vi "main.vi"() -> ()   [LabVIEW 2019]
uses:
  <vilib>/Utility/sysdir.llb/System Directory Type.ctl
  <vilib>/Platform/browser.llb/Open URL in Default Browser (string).vi
  <vilib>/Utility/cursorutil.llb/Set Cursor (Icon Pict).vi
  <vilib>/regexp/Match Regular Expression.xnode
  lib/libSimulationControl/libSimulationControl.lvlib
panel:
  out "Impressum":string
  out "Running?":bool
  in  "Help Button":bool
  in  "Break":bool
  in  "Plot":bool
  in  "Stop Button":bool
  in  "Pause Button":bool
  in  "Run":bool
  in  "Tab Control":T1(tab)
  out "Active element":string
  out "Iteration":i32
  out "Plant structure":string
  out "Simulation log":string
  in  "Auto Scroll":bool
  in  "Reset":bool
  in  "Uncouple":bool
  out "Working directory":path
  out "Runtime":dbl
  in  "Console":bool
  out "Runtime":string
  in  "Env. Clear":bool
  out "Env. Structure":string
  in  "Load Env":bool
  out "Environtment ready?":bool
  in  "Create Env":bool
  in  "Environtment Dir":path
  in  "Environment Tree":string(tree)
  out "Reactor Legend":picture
  in  "Show legend":bool
  out "Feedback?":bool
  out "Methane?":bool
  out "Storage?":bool
  out "#Hydrolysis":dbl
  out "Plant":picture
  in  "Reactor State":string(combo)="STRUCT_1_STAGE.vi"
  in  "Hydrolysis specification":path
  in  "Methane specification":path
  in  "Auto cleanup?":bool
  in  "Endtime":dbl
  in  "Starttime":dbl
  in  "Edit Methane":bool
  in  "Edit Hydro":bool
  in  "Simulation file":path
  out "#Reactors":i32
  in  "Inflow fractions":T2(array[cluster]) {"Vertical Pointer Slide" scale=0.0..100.0 scale format="%.0f%"}
  in  "Hydrolysis PH":cluster{"Meter":dbl, "String":string}[][](array[cluster]) {"Meter" scale=0.0..14.0}
  in  "Load Feeding":bool
  in  "Save Feeding":bool
  out "Valid stamp?":bool
  out "Next timestep":dbl
  in  "Reactor":string(combo)
  in  "Delete":bool
  in  "Add timestamp":string[](array[string])
  in  "Add":bool
  in  "Feeding table":i32(listbox)
  out "timetable":string
  # "Biogas simulation Control"
  # "Before you start the simulation you need to set up a working environment.\nThe environment will be for the chosen reactor structure only."
  # "If you want the hydrolysis reactors to start with different initial values, you need to set up a working environtment first."
  # "Change the proportions at which the methane outflow will \nbe fed back into the hydrolysis reactors:"
  # "Add feeding hours and amount for a hydrolysis reactor."
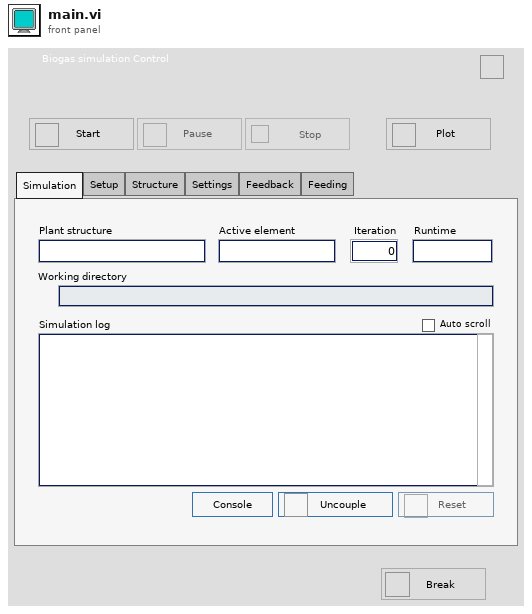
[diagram p1: front panel]
types:
  T1 = enum32{"Simulation", "Setup", "Structure", "Settings", "Feedback", "Feeding"}
  T2 = cluster{"Vertical Pointer Slide":i32, "String":string}[]
  T3 = typedef "System Directory Type.ctl" = i32
  T4 = enum8{"Enabled", "Disabled", "Disabled and Grayed Out"}
  T5 = typedef "LVPoint32TypeDef.ctl" = cluster{"Horizontal":i32, "Vertical":i32}
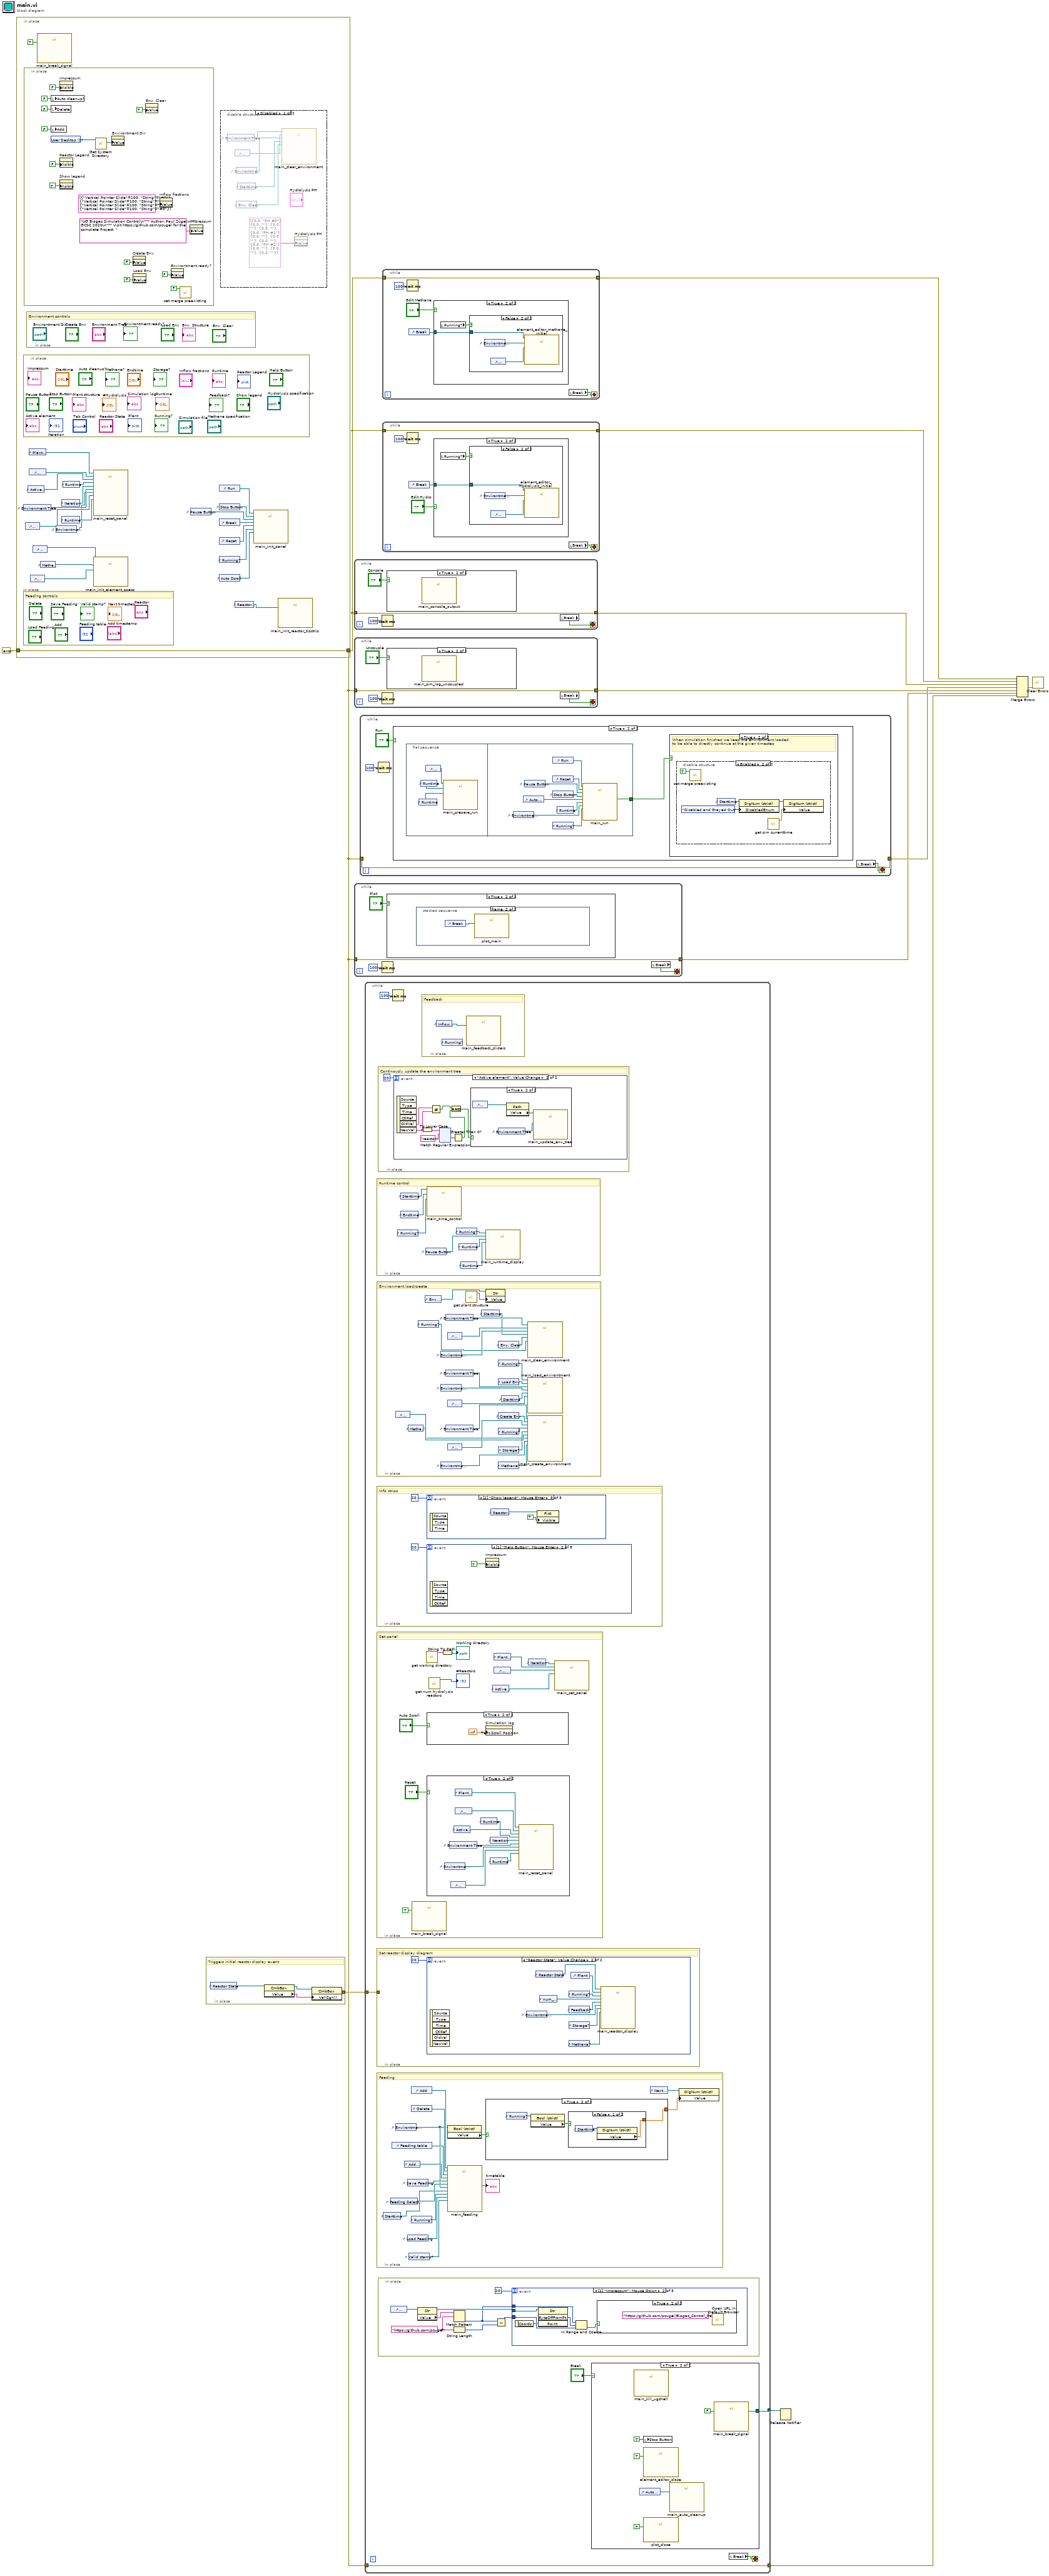
[diagram p0: block diagram]
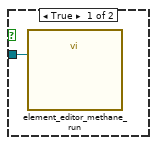
[diagram p3: hidden frame]
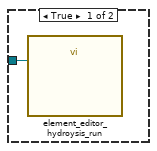
[diagram p5: hidden frame]
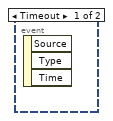
[diagram p8: hidden frame]
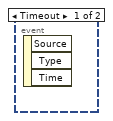
[diagram p10: hidden frame]
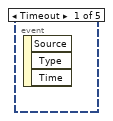
[diagram p11: hidden frame]
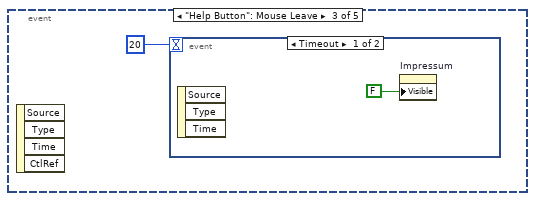
[diagram p12: hidden frame]
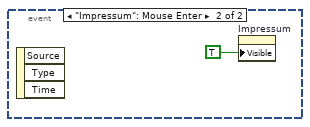
[diagram p13: hidden frame]
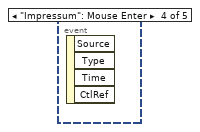
[diagram p14: hidden frame]
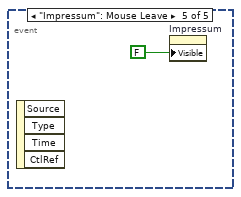
[diagram p15: hidden frame]
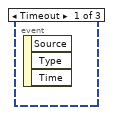
[diagram p16: hidden frame]
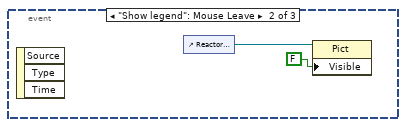
[diagram p17: hidden frame]
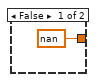
[diagram p20: hidden frame]
diagram:
  n1 = in-place {
    in-place-border: [w34] -> w5
    in-place-border: errorcluster {"status"=FALSE, "code"=0, "source"=""} ("error constant") -> [w34]
    n2 = in-place {
    }
    n3 = control-ref of="Environment Tree"() -> (w17:refnum<vi>)
    n4 = in-place {
      # "Feeding controls"
    }
    n5 = in-place {
      w46 = T3 1 items=["User Home"=0, "User Desktop"=1, "User Documents"=2, "User Application Data"=3, "User Preferences"=4, "User Temporary"=5, "Public Documents"=6, "Public Application Data"=7, "Public Preferences"=8, "Public Cache"=13, "System Core Libraries"=9, "System Installed Libraries"=10, "Application Files"=11, "Boot Volume Root"=12] ("system directory type")
      n6 = local write "Auto cleanup?"(FALSE ("Auto Cleanup?")) -> ()
      n7 = local write "Delete"(FALSE ("Delete")) -> ()
      n8 = local write "Add"(FALSE ("Add")) -> ()
      n9 = property on="Impressum" class="Str"("Visible"=FALSE) -> ()  [unwired: 2 in, 2 out]
      n10 = property on="Reactor Legend" class="Pict"("Visible"=FALSE) -> ()  [unwired: 2 in, 2 out]
      n11 = property on="Show legend" class="Bool"("Visible"=TRUE) -> ()  [unwired: 2 in, 2 out]
      n12 = call <vilib>:"Get System Directory.vi"("system directory type"=w46) -> ("system directory"=w47:path)  [unwired: 10 in]
      n13 = property on="Environtment Dir" class="Path"("Value"=w47) -> ()  [unwired: 2 in, 2 out]
      n14 = property on="Create Env" class="Bool (strict)"("Value"=FALSE ("Create Env")) -> ()  [unwired: 2 in, 2 out]
      n15 = property on="Load Env" class="Bool (strict)"("Value"=FALSE ("Load Env")) -> ()  [unwired: 2 in, 2 out]
      n16 = property on="Env. Clear" class="Bool (strict)"("Value"=TRUE ("Env. Clear")) -> ()  [unwired: 2 in, 2 out]
      n17 = property on="Inflow fractions" class="Arr (strict)"("Value"=T2 [{"Vertical Pointer Slide"=100, "String"="#0"}, {"Vertical Pointer Slide"=100, "String"="#1"}, {"Vertical Pointer Slide"=100, "String"="#2"}, {"Vertical Pointer Slide"=100, "String"="#3"}] ("Inflow fractions")) -> ()  [unwired: 2 in, 2 out]
      n18 = property on="Environtment ready?" class="Bool (strict)"("Value"=FALSE ("Environtment ready?")) -> ()  [unwired: 2 in, 2 out]
      n19 = call "set merge preexisting.vi"("merge"=FALSE) -> ()  [unwired: 10 in, 1 out]
      n20 = property on="Impressum" class="Str"("Value"="UG Biogas Simulation Control\n*** Author: Paul Zügel\n*** GCSC 2020\n*** Visit https://github.com/pzugel for the complete Project  " ("String")) -> ()  [unwired: 2 in, 2 out]
    }
    n21 = control-ref of="Environtment Dir"() -> (w18:refnum<vi>)
    n22 = in-place {
      # "Environment controls"
    }
    n23 = control-ref of="Active element"() -> (w32:refnum<vi>)
    n24 = control-ref of="Plant structure"() -> (w30:refnum<vi>)
    n25 = control-ref of="Simulation log"() -> (w31:refnum<vi>)
    n26 = control-ref of="Simulation file"() -> (w20:refnum<vi>)
    n27 = control-ref of="Hydrolysis specification"() -> (w14:refnum<vi>)
    n28 = call "main_break_signal.vi"("Keep Running?"=TRUE ("Checkbox")) -> ()  [unwired: 10 in, 1 out]
    n29 = control-ref of="Methane specification"() -> (w13:refnum<vi>)
    n30 = control-ref of="Environtment ready?"() -> (w16:refnum<vi>)
    n31 = control-ref of="Iteration"() -> (w33:refnum<vi>)
    n32 = control-ref of="Runtime"() -> (w21:refnum<vi>)
    n33 = control-ref of="Runtime"() -> (w19:refnum<vi>)
    n34 = call "main_reset_panel.vi"("Env ready?"=w16, "Envi. Tree"=w17, "Env. Directory"=w18, "Iteration"=w33, "Runtime"=w21, "Runtime (string)"=w19, "Active Element"=w32, "Simulation Log"=w31, "Plant Structure"=w30) -> ()  [unwired: 3 in]
    n35 = call "main_init_element_specs.vi"("Simulation"=w20, "Methane"=w13, "Hydrolyse"=w14) -> ()  [unwired: 9 in]
    n36 = control-ref of="Pause Button"() -> (w23:refnum<vi>)
    n37 = control-ref of="Run"() -> (w29:refnum<vi>)
    n38 = control-ref of="Stop Button"() -> (w24:refnum<vi>)
    n39 = control-ref of="Break"() -> (w27:refnum<vi>)
    n40 = control-ref of="Reset"() -> (w28:refnum<vi>)
    n41 = control-ref of="Running?"() -> (w22:refnum<vi>)
    n42 = control-ref of="Auto Scroll"() -> (w26:refnum<vi>)
    n43 = disable-structure shown="Disabled" {
      frame Disabled {
        n44 = control-ref of="Environment Tree"() -> (w40:refnum<vi>)
        n45 = control-ref of="Environtment Dir"() -> (w39:refnum<vi>)
        n46 = control-ref of="Environtment ready?"() -> (w38:refnum<vi>)
        n47 = control-ref of="Env. Clear"() -> (w36:refnum<vi>)
        n48 = control-ref of="Starttime"() -> (w37:refnum<vi>)
        n49 = call "main_clear_environment.vi"("Env. Clear"=w36, "Starttime"=w37, "Env. ready?"=w38, "Env. Dir"=w39, "Env. Tree"=w40) -> ()  [unwired: 7 in]
        n50 = property on="Hydrolysis PH" class="Arr (strict)"("Value"=cluster{"Meter":dbl, "String":string}[][] [[{"Meter"=0.0, "String"="PH #0"}, {"Meter"=0.0, "String"=""}, {"Meter"=0.0, "String"=""}, {"Meter"=0.0, "String"=""}], [{"Meter"=0.0, "String"="PH #1"}, {"Meter"=0.0, "String"=""}, {"Meter"=0.0, "String"=""}, {"Meter"=0.0, "String"=""}], [{"Meter"=0.0, "String"="PH #2"}, {"Meter"=0.0, "String"=""}, {"Meter"=0.0, "String"=""}, {"Meter"=0.0, "String"=""}]] ("Hydrolysis PH")) -> ()  [unwired: 2 in, 2 out]
      }
      frame Enabled {
      }
    }
    n51 = control-ref of="Reactor Legend"() -> (w15:refnum<vi>)
    n52 = call "main_init_panel.vi"("Running?"=w22, "Reset"=w28, "Auto Scroll"=w26, "Break Button"=w27, "Pause Button"=w23, "Stop Button"=w24, "Run"=w29) -> ()  [unwired: 5 in]
    n53 = call "main_init_reactor_tipstrip.vi"("Reactor legend"=w15) -> ()  [unwired: 11 in]
  }
  n54 = in-place {
    in-place-border: [w56] -> w1
    # "Triggers initial reactor display event"
    n55 = control-ref of="Reactor State"() -> (w59:refnum<vi>)
    n56 = property class="CmbBox"(reference=w59) -> (reference out=w57:refnum<vi>, "Value"=w58:string)  [unwired: 1 in, 1 out]
    n57 = property class="CmbBox"(reference=w57, "Val(Sgnl)"=w58) -> (error out=w56:errorcluster)  [unwired: 1 in, 1 out]
  }
  n58 = while {
    tunnel: w5 -> [w62]
    tunnel: [w62] -> w6
    stop <- w60 stop-if-true
    n59 = Wait (ms)(milliseconds to wait=u32 100) -> ()  [unwired: 1 out]
    n60 = case shown="True" "Console" {
      frame False {
      }
      frame True {
        n61 = call "main_console_output.vi"() -> ()  [unwired: 12 in]
      }
    }
    n62 = local read "Break"() -> (w60:bool)
  }
  n63 = while {
    tunnel: w5 -> [w66]
    tunnel: [w66] -> w7
    stop <- w64 stop-if-true
    n64 = Wait (ms)(milliseconds to wait=u32 100) -> ()  [unwired: 1 out]
    n65 = case shown="True" "Uncouple" {
      frame False {
      }
      frame True {
        n66 = call "main_sim_log_uncoupled.vi"() -> ()  [unwired: 12 in]
      }
    }
    n67 = local read "Break"() -> (w64:bool)
  }
  n68 = while {
    tunnel: w5 -> [w70]
    tunnel: [w70] -> w10
    stop <- w68 stop-if-true
    n69 = Wait (ms)(milliseconds to wait=u32 100) -> ()  [unwired: 1 out]
    n70 = case shown="True" "Plot" {
      frame False {
      }
      frame True {
        n71 = stacked-sequence {
          frame #0 {
            n72 = call "plot_close.vi"("Close?"=TRUE) -> ()  [unwired: 11 in]
          }
          frame #1 {
            n73 = control-ref of="Break"() -> (w73:refnum<vi>)
            n74 = call "plot_main.vi"("Break"=w73) -> ()  [unwired: 11 in]
          }
        }
      }
    }
    n75 = local read "Break"() -> (w68:bool)
  }
  n76 = while {
    tunnel: w5 -> [w77]
    tunnel: [w77] -> w11
    stop <- w75 stop-if-true
    n77 = Wait (ms)(milliseconds to wait=u32 100) -> ()  [unwired: 1 out]
    n78 = case shown="True" "Run" {
      frame False {
        n79 = property on="Run" class="Bool"("DisabledEnum"=T4."Enabled" ("Disabled")) -> ()  [unwired: 2 in, 2 out]
        n80 = property on="Stop Button" class="Bool (strict)"("DisabledEnum"=T4."Disabled and Grayed Out" ("Disabled")) -> ()  [unwired: 2 in, 2 out]
        n81 = property on="Pause Button" class="Bool (strict)"("DisabledEnum"=T4."Disabled and Grayed Out" ("Disabled")) -> ()  [unwired: 2 in, 2 out]
      }
      frame True {
        n82 = flat-sequence {
          tunnel: [w96] -> w81
          frame #0 {
            n83 = control-ref of="Runtime"() -> (w95:refnum<vi>)
            n84 = control-ref of="Runtime"() -> (w94:refnum<vi>)
            n85 = control-ref of="Environtment Dir"() -> (w93:refnum<vi>)
            n86 = call "main_prepare_run.vi"("Runtime"=w95, "Runtime String"=w94, "Env. Dir"=w93) -> ()  [unwired: 9 in]
          }
          frame #1 {
            n87 = control-ref of="Environtment ready?"() -> (w104:refnum<vi>)
            n88 = control-ref of="Auto cleanup?"() -> (w103:refnum<vi>)
            n89 = control-ref of="Pause Button"() -> (w100:refnum<vi>)
            n90 = control-ref of="Run"() -> (w98:refnum<vi>)
            n91 = control-ref of="Reset"() -> (w102:refnum<vi>)
            n92 = control-ref of="Stop Button"() -> (w99:refnum<vi>)
            n93 = control-ref of="Running?"() -> (w101:refnum<vi>)
            n94 = control-ref of="Runtime"() -> (w97:refnum<vi>)
            n95 = call "main_run.vi"("Runtime String"=w97, "Env ready?"=w104, "Cleanup?"=w103, "Running?"=w101, "Stop Button"=w99, "Pause Button"=w100, "Reset"=w102, "Run"=w98) -> ("OK?"=w96:bool)  [unwired: 3 in]
          }
        }
        n96 = case shown="True" w81 {
          frame False {
          }
          frame True {
            # "When simulation finished we keep the environment loaded\nto be able to directly continue at the given timestep"
            n97 = disable-structure shown="Enabled" {
              frame Disabled {
                n98 = control-ref of="Env. Clear"() -> (w86:refnum<vi>)
                n99 = property class="Bool (strict)"(reference=w86, "Value"=TRUE) -> (reference out=w87:refnum<vi>)  [unwired: 1 in, 1 out]
                n100 = control-ref of="Environtment ready?"() -> (w85:refnum<vi>)
                n101 = control-ref of="Environment Tree"() -> (w83:refnum<vi>)
                n102 = control-ref of="Environtment Dir"() -> (w84:refnum<vi>)
                n103 = call "main_clear_environment.vi"("Env. Clear"=w87, "Env. ready?"=w85, "Env. Dir"=w84, "Env. Tree"=w83) -> ()  [unwired: 8 in]
              }
              frame Enabled {
                n104 = call "set merge preexisting.vi"("merge"=TRUE) -> ()  [unwired: 10 in, 1 out]
                n105 = control-ref of="Starttime"() -> (w91:refnum<vi>)
                n106 = property class="DigNum (strict)"(reference=w91, "DisabledEnum"=T4."Disabled and Grayed Out" ("Disabled")) -> (reference out=w88:refnum<vi>)  [unwired: 1 in, 1 out]
                n107 = call "get sim currenttime.vi"() -> ("current_time"=w89:dbl)  [unwired: 10 in, 1 out]
                n108 = property class="DigNum (strict)"(reference=w88, "Value"=w89) -> ()  [unwired: 1 in, 2 out]
              }
            }
          }
        }
      }
    }
    n109 = local read "Break"() -> (w75:bool)
  }
  n110 = while {
    tunnel: w5 -> [w110]
    tunnel: [w110] -> w9
    tunnel: [w108] -> w8
    tunnel: w1 -> [w105]
    stop <- w106 stop-if-true
    n111 = in-place {
      # "Runtime control"
      n112 = control-ref of="Running?"() -> (w242:refnum<vi>)
      n113 = control-ref of="Starttime"() -> (w244:refnum<vi>)
      n114 = control-ref of="Endtime"() -> (w243:refnum<vi>)
      n115 = control-ref of="Pause Button"() -> (w239:refnum<vi>)
      n116 = call "main_time_control.vi"("Running?"=w242, "Endtime"=w243, "Starttime"=w244) -> ()  [unwired: 9 in]
      n117 = control-ref of="Running?"() -> (w238:refnum<vi>)
      n118 = control-ref of="Runtime"() -> (w240:refnum<vi>)
      n119 = control-ref of="Runtime"() -> (w241:refnum<vi>)
      n120 = call "main_runtime_display.vi"("Runtime (string)"=w241, "Runtime"=w240, "Pause Button"=w239, "Running?"=w238) -> ()  [unwired: 8 in]
    }
    n121 = in-place {
      # "Environment load/create"
      n122 = control-ref of="Hydrolysis specification"() -> (w287:refnum<vi>)
      n123 = control-ref of="Methane specification"() -> (w286:refnum<vi>)
      n124 = control-ref of="Running?"() -> (w285:refnum<vi>)
      n125 = control-ref of="Env. Structure"() -> (w297:refnum<vi>)
      n126 = control-ref of="Environtment ready?"() -> (w293:refnum<vi>)
      n127 = control-ref of="Environtment ready?"() -> (w296:refnum<vi>)
      n128 = control-ref of="Environtment ready?"() -> (w301:refnum<vi>)
      n129 = control-ref of="Environment Tree"() -> (w291:refnum<vi>)
      n130 = control-ref of="Environment Tree"() -> (w298:refnum<vi>)
      n131 = control-ref of="Environment Tree"() -> (w307:refnum<vi>)
      n132 = control-ref of="Environtment Dir"() -> (w292:refnum<vi>)
      n133 = control-ref of="Environtment Dir"() -> (w295:refnum<vi>)
      n134 = control-ref of="Environtment Dir"() -> (w305:refnum<vi>)
      n135 = call "get plant structure.vi"() -> ("function return"=w289:string)  [unwired: 10 in, 1 out]
      n136 = control-ref of="Starttime"() -> (w288:refnum<vi>)
      n137 = property class="Str"(reference=w297, "Value"=w289) -> ()  [unwired: 1 in, 2 out]
      n138 = control-ref of="Env. Clear"() -> (w294:refnum<vi>)
      n139 = control-ref of="Running?"() -> (w300:refnum<vi>)
      n140 = control-ref of="Load Env"() -> (w299:refnum<vi>)
      n141 = control-ref of="Create Env"() -> (w306:refnum<vi>)
      n142 = control-ref of="Running?"() -> (w304:refnum<vi>)
      n143 = control-ref of="Storage?"() -> (w303:refnum<vi>)
      n144 = control-ref of="Methane?"() -> (w302:refnum<vi>)
      n145 = control-ref of="Starttime"() -> (w290:refnum<vi>)
      n146 = call "main_clear_environment.vi"("Env. Clear"=w294, "Running?"=w285, "Starttime"=w288, "Env. ready?"=w293, "Env. Dir"=w292, "Env. Tree"=w291) -> ()  [unwired: 6 in]
      n147 = call "main_load_environtment.vi"("Starttime"=w290, "Env. Dir"=w295, "Env. Ready?"=w296, "Environtment Tree"=w298, "Load Env"=w299, "Running?"=w300) -> ()  [unwired: 6 in]
      n148 = call "main_create_environment.vi"("Meth. Path"=w286, "Hydr. Path"=w287, "Ready?"=w301, "Storage?"=w303, "Methane?"=w302, "Running?"=w304, "Directory"=w305, "Create"=w306, "Environtment Tree"=w307) -> ()  [unwired: 3 in]
    }
    n149 = in-place {
      # "Info strips"
      n150 = event shown="[2] \"Show legend\": Mouse Enter" {
        selector: _ -> [_ _ _]
        dyn-events: _ -> [_ _ _]
        timeout: 20 -> [_ _ _]
        event Timeout {
          n151 = event-data() -> ()  [unwired: 1 in, 3 out]
        }
        event "Show legend": Mouse Leave {
          n152 = event-data() -> ()  [unwired: 1 in, 3 out]
          n153 = control-ref of="Reactor Legend"() -> (w262:refnum<vi>)
          n154 = property class="Pict"(reference=w262, "Visible"=FALSE) -> ()  [unwired: 1 in, 2 out]
        }
        event "Show legend": Mouse Enter {
          n155 = event-data() -> ()  [unwired: 1 in, 3 out]
          n156 = control-ref of="Reactor Legend"() -> (w264:refnum<vi>)
          n157 = property class="Pict"(reference=w264, "Visible"=TRUE) -> ()  [unwired: 1 in, 2 out]
        }
      }
      n158 = event shown="[1] \"Help Button\": Mouse Enter" {
        selector: _ -> [_ _ _ _ _]
        dyn-events: _ -> [_ _ _ _ _]
        timeout: 20 -> [_ _ _ _ _]
        event Timeout {
          n159 = event-data() -> ()  [unwired: 1 in, 3 out]
        }
        event "Help Button": Mouse Enter {
          n160 = event-data() -> ()  [unwired: 1 in, 4 out]
          n161 = property on="Impressum" class="Str"("Visible"=TRUE) -> ()  [unwired: 2 in, 2 out]
        }
        event "Help Button": Mouse Leave {
          n162 = event-data() -> ()  [unwired: 1 in, 4 out]
          n163 = event shown="[0] Timeout" {
            selector: _ -> [_ _]
            dyn-events: _ -> [_ _]
            timeout: 20 -> [_ _]
            event Timeout {
              n164 = event-data() -> ()  [unwired: 1 in, 3 out]
              n165 = property on="Impressum" class="Str"("Visible"=FALSE) -> ()  [unwired: 2 in, 2 out]
            }
            event "Impressum": Mouse Enter {
              n166 = event-data() -> ()  [unwired: 1 in, 3 out]
              n167 = property on="Impressum" class="Str"("Visible"=TRUE) -> ()  [unwired: 2 in, 2 out]
            }
          }
        }
        event "Impressum": Mouse Enter {
          n168 = event-data() -> ()  [unwired: 1 in, 4 out]
        }
        event "Impressum": Mouse Leave {
          n169 = event-data() -> ()  [unwired: 1 in, 4 out]
          n170 = property on="Impressum" class="Str"("Visible"=FALSE) -> ()  [unwired: 2 in, 2 out]
        }
      }
    }
    n171 = in-place {
      # "Set panel"
      n172 = call "main_break_signal.vi"("Keep Running?"=TRUE) -> ()  [unwired: 10 in, 1 out]
      n173 = call "get working directory.vi"() -> ("function return"=w274:string)  [unwired: 10 in, 1 out]
      n174 = case shown="True" "Auto Scroll" {
        frame False {
        }
        frame True {
          n175 = property on="Simulation log" class="Str"("Text.Scroll Position"=inf) -> ()  [unwired: 2 in, 2 out]
        }
      }
      n176 = case shown="True" "Reset" {
        frame False {
        }
        frame True {
          n177 = control-ref of="Environtment ready?"() -> (w276:refnum<vi>)
          n178 = control-ref of="Environment Tree"() -> (w277:refnum<vi>)
          n179 = control-ref of="Environtment Dir"() -> (w278:refnum<vi>)
          n180 = control-ref of="Active element"() -> (w282:refnum<vi>)
          n181 = control-ref of="Plant structure"() -> (w283:refnum<vi>)
          n182 = control-ref of="Simulation log"() -> (w280:refnum<vi>)
          n183 = control-ref of="Runtime"() -> (w275:refnum<vi>)
          n184 = control-ref of="Iteration"() -> (w281:refnum<vi>)
          n185 = control-ref of="Runtime"() -> (w279:refnum<vi>)
          n186 = call "main_reset_panel.vi"("Env ready?"=w276, "Envi. Tree"=w277, "Env. Directory"=w278, "Iteration"=w281, "Runtime"=w279, "Runtime (string)"=w275, "Active Element"=w282, "Simulation Log"=w280, "Plant Structure"=w283) -> ()  [unwired: 3 in]
        }
      }
      n187 = call "get num hydrolysis reactors.vi"() -> ("function return"=→"#Reactors":i32)  [unwired: 10 in, 1 out]
      n188 = String To Path(string=w274) -> (path=→"Working directory":path)
      n189 = control-ref of="Active element"() -> (w268:refnum<vi>)
      n190 = control-ref of="Plant structure"() -> (w266:refnum<vi>)
      n191 = control-ref of="Simulation log"() -> (w267:refnum<vi>)
      n192 = control-ref of="Iteration"() -> (w265:refnum<vi>)
      n193 = call "main_set_panel.vi"("Active Element"=w268, "Simulation Log"=w267, "Plant Structure"=w266, "Iteration"=w265) -> ()  [unwired: 8 in]
    }
    n194 = in-place {
      in-place-border: w105 -> [_]
      # "Set reactor display diagram"
      n195 = event shown="[1] \"Reactor State\": Value Change" {
        selector: _ -> [_ _]
        dyn-events: _ -> [_ _]
        timeout: 20 -> [_ _]
        event Timeout {
          n196 = event-data() -> ()  [unwired: 1 in, 3 out]
        }
        event "Reactor State": Value Change {
          n197 = event-data() -> ()  [unwired: 1 in, 6 out]
          n198 = control-ref of="Environtment ready?"() -> (w253:refnum<vi>)
          n199 = control-ref of="Reactor State"() -> (w246:refnum<vi>)
          n200 = control-ref of="num_Hydrolysis"() -> (w249:refnum<vi>)
          n201 = control-ref of="Running?"() -> (w248:refnum<vi>)
          n202 = control-ref of="Feedback?"() -> (w252:refnum<vi>)
          n203 = control-ref of="Storage?"() -> (w250:refnum<vi>)
          n204 = control-ref of="Methane?"() -> (w251:refnum<vi>)
          n205 = control-ref of="Plant"() -> (w247:refnum<vi>)
          n206 = call "main_reactor_display.vi"("Env. Ready?"=w253, "Storage?"=w250, "Feedback?"=w252, "Methane?"=w251, "#Hydrolysis"=w249, "Running?"=w248, "Plant Picture"=w247, "Reactor State"=w246) -> ()  [unwired: 4 in]
        }
      }
    }
    n207 = in-place {
      # "Feeding"
      n208 = control-ref of="Starttime"() -> (w308:refnum<vi>)
      n209 = control-ref of="Feeding Select Reactor"() -> (w314:refnum<vi>)
      n210 = control-ref of="Feeding table"() -> (w322:refnum<vi>)
      n211 = control-ref of="Environtment ready?"() -> (w309:refnum<vi>)
      n212 = control-ref of="Add timestamp"() -> (w321:refnum<vi>)
      n213 = control-ref of="Save Feeding"() -> (w316:refnum<vi>)
      n214 = control-ref of="Load Feeding"() -> (w315:refnum<vi>)
      n215 = control-ref of="Valid stamp?"() -> (w318:refnum<vi>)
      n216 = control-ref of="Add"() -> (w320:refnum<vi>)
      n217 = control-ref of="Delete"() -> (w319:refnum<vi>)
      n218 = control-ref of="Running?"() -> (w312:refnum<vi>)
      n219 = call "main_feeding.vi"("Env. Ready?"=w309, "Starttime"=w308, "Running?"=w312, "Selector"=w314, "Load"=w315, "Save"=w316, "Valid?"=w318, "New Element"=w321, "Feeding"=w322, "Delete"=w319, "Add"=w320) -> ("timetable"=→"timetable":string)
      n220 = property class="Bool (strict)"(reference=w309) -> ("Value"=w313:bool)  [unwired: 1 in, 2 out]
      n221 = case shown="True" w313 {
        tunnel: [nan w324] -> w311
        frame False {
        }
        frame True {
          n222 = control-ref of="Running?"() -> (w326:refnum<vi>)
          n223 = property class="Bool (strict)"(reference=w326) -> ("Value"=w325:bool)  [unwired: 1 in, 2 out]
          n224 = case shown="False" w325 {
            tunnel: [w327 w329] -> w324
            frame False {
              n225 = control-ref of="Starttime"() -> (w328:refnum<vi>)
              n226 = property class="DigNum (strict)"(reference=w328) -> ("Value"=w327:dbl)  [unwired: 1 in, 2 out]
            }
            frame True {
              n227 = call "get sim currenttime.vi"() -> ("current_time"=w330:dbl)  [unwired: 10 in, 1 out]
              n228 = Increment(x=w330) -> (x+1=w329:dbl)
            }
          }
        }
      }
      n229 = control-ref of="Next timestep"() -> (w310:refnum<vi>)
      n230 = property class="DigNum (strict)"(reference=w310, "Value"=w311) -> ()  [unwired: 1 in, 2 out]
    }
    n231 = in-place {
      # "Continously update the environment tree"
      n232 = event shown="[1] \"Active element\": Value Change" {
        selector: _ -> [_ _]
        dyn-events: _ -> [_ _]
        timeout: 20 -> [_ _]
        event Timeout {
          n233 = event-data() -> ()  [unwired: 1 in, 3 out]
        }
        event "Active element": Value Change {
          n234 = event-data() -> ("OldVal"=w116:string, "NewVal"=w115:string)  [unwired: 1 in, 4 out]
          n235 = To Lower Case(string=w115) -> (all lower case string=w118:string)
          n236 = Not Equal?(x=w116, y=w115) -> (x != y?=w114:bool)
          n237 = xnode "Match Regular Expression"("input string"=w118, "regular expression"="reactor") -> ("offset past match"=w119:i32)  [unwired: 4 in, 4 out]
          n238 = Greater Than 0?(x=w119) -> (x > 0?=w113:bool)
          n239 = And(x=w114, y=w113) -> (x .and. y?=w112:bool)
          n240 = case shown="True" w112 {
            frame False {
            }
            frame True {
              n241 = control-ref of="Environtment Dir"() -> (w121:refnum<vi>)
              n242 = control-ref of="Environment Tree"() -> (w122:refnum<vi>)
              n243 = property class="Path"(reference=w121) -> ("Value"=w120:path)  [unwired: 1 in, 2 out]
              n244 = call "main_update_env_tree.vi"("Env. Tree"=w122, "Env_path"=w120) -> ()  [unwired: 10 in]
            }
          }
        }
      }
    }
    n245 = in-place {
      w334 = "https://github.com/pzugel" ("regular expression")
      n246 = control-ref of="Impressum"() -> (w331:refnum<vi>)
      n247 = property class="Str"(reference=w331) -> (reference out=w338:refnum<vi>, "Value"=w333:string)  [unwired: 1 in, 1 out]
      n248 = Match Pattern(string=w333, regular expression=w334) -> (offset past match=w336:i32)  [unwired: 1 in, 3 out]
      n249 = String Length(string=w334) -> (length=w332:i32)
      n250 = Subtract(x=w336, y=w332) -> (x-y=w335:i32)
      n251 = event shown="[1] \"Impressum\": Mouse Down" {
        selector: _ -> [_ _ _]
        dyn-events: _ -> [_ _ _]
        timeout: 20 -> [_ _ _]
        tunnel: w335 -> [_ w342 w349]
        tunnel: w336 -> [_ w343 w350]
        tunnel: w338 -> [_ w340 w347]
        event Timeout {
          n252 = event-data() -> ()  [unwired: 1 in, 3 out]
        }
        event "Impressum": Mouse Down {
          n253 = event-data() -> ("Coords"=w339:T5)  [unwired: 1 in]
          n254 = invoke class="Str" method="ByteOffFromPt"(reference=w340, "Point"=w339) -> ("ByteOffFromPt"=w344:i32)  [unwired: 2 in, 3 out]
          n255 = In Range and Coerce(upper limit=w343, x=w344, lower limit=w342) -> (In Range?=w341:bool)  [unwired: 1 out]
          n256 = case shown="True" w341 {
            frame False {
            }
            frame True {
              n257 = call-poly <vilib>:"Open URL in Default Browser.vi"("URL"="https://github.com/pzugel/Biogas_Control_Panel") -> ()  [unwired: 5 in, 2 out]
            }
          }
        }
        event "Impressum": Mouse Move {
          n258 = event-data() -> ("Coords"=w346:T5)  [unwired: 1 in]
          n259 = invoke class="Str" method="ByteOffFromPt"(reference=w347, "Point"=w346) -> ("ByteOffFromPt"=w351:i32)  [unwired: 2 in, 3 out]
          n260 = In Range and Coerce(upper limit=w350, x=w351, lower limit=w349) -> (In Range?=w348:bool)  [unwired: 1 out]
          n261 = case shown="True" w348 {
            frame False {
              n262 = call-poly <vilib>:"Set Cursor.vi"("icon"=u16 1) -> ()  [unwired: 9 in, 2 out]
            }
            frame True {
              n263 = call-poly <vilib>:"Set Cursor.vi"("icon"=u16 6) -> ()  [unwired: 9 in, 2 out]
            }
          }
        }
      }
    }
    n264 = Wait (ms)(milliseconds to wait=u32 100) -> ()  [unwired: 1 out]
    n265 = in-place {
      # "Feedback"
      n266 = control-ref of="Inflow fractions"() -> (w237:refnum<vi>)
      n267 = control-ref of="Running?"() -> ()  [unwired: 1 out]
      n268 = call "main_feedback_sliders.vi"("Inflow fractions"=w237) -> ()  [unwired: 11 in]
    }
    n269 = case shown="True" "Break" {
      tunnel: [w355 w357] -> w108
      frame False {
        n270 = call "main_break_signal.vi"("Keep Running?"=TRUE ("Checkbox")) -> ("Break Notifier"=w355:refnum<notifier>)  [unwired: 10 in]
      }
      frame True {
        n271 = call "main_kill_ugshell.vi"() -> ()  [unwired: 12 in]
        n272 = control-ref of="Auto cleanup?"() -> (w356:refnum<vi>)
        n273 = local write "Stop Button"(TRUE ("Stop Button")) -> ()
        n274 = call "element_editor_close.vi"("Close?"=TRUE ("Checkbox")) -> ()  [unwired: 11 in]
        n275 = call "plot_close.vi"("Close?"=TRUE) -> ()  [unwired: 11 in]
        n276 = call "main_auto_cleanup.vi"("Cleanup?"=w356) -> ()  [unwired: 11 in]
        n277 = call "main_break_signal.vi"("Keep Running?"=FALSE ("Checkbox")) -> ("Break Notifier"=w357:refnum<notifier>)  [unwired: 10 in]
      }
    }
    n278 = local read "Break"() -> (w106:bool)
  }
  n279 = while {
    tunnel: w5 -> [w365]
    tunnel: [w365] -> w3
    stop <- w362 stop-if-true
    n280 = Wait (ms)(milliseconds to wait=u32 100) -> ()  [unwired: 1 out]
    n281 = control-ref of="Break"() -> (w363:refnum<vi>)
    n282 = case shown="True" "Edit Methane" {
      tunnel: w363 -> [_ w368]
      frame False {
      }
      frame True {
        n283 = local read "Running?"() -> (w367:bool)
        n284 = case shown="False" w367 {
          tunnel: w368 -> [w369 w372]
          frame True {
            n285 = call "element_editor_methane_run.vi"("Break"=w369) -> ()  [unwired: 11 in]
          }
          frame False {
            n286 = control-ref of="Environtment ready?"() -> (w371:refnum<vi>)
            n287 = control-ref of="Environtment Dir"() -> (w370:refnum<vi>)
            n288 = call "element_editor_methane_initial.vi"("Env. Dir"=w370, "Env. Ready?"=w371, "Break"=w372) -> ()  [unwired: 9 in]
          }
        }
      }
    }
    n289 = local read "Break"() -> (w362:bool)
  }
  n290 = while {
    tunnel: w5 -> [w377]
    tunnel: [w377] -> w4
    stop <- w373 stop-if-true
    n291 = Wait (ms)(milliseconds to wait=u32 100) -> ()  [unwired: 1 out]
    n292 = control-ref of="Break"() -> (w374:refnum<vi>)
    n293 = case shown="True" "Edit Hydro" {
      tunnel: w374 -> [_ w378]
      frame False {
      }
      frame True {
        n294 = local read "Running?"() -> (w379:bool)
        n295 = case shown="False" w379 {
          tunnel: w378 -> [w380 w381]
          frame True {
            n296 = call "element_editor_hydroysis_run.vi"("Break"=w380) -> ()  [unwired: 11 in]
          }
          frame False {
            n297 = control-ref of="Environtment ready?"() -> (w383:refnum<vi>)
            n298 = control-ref of="Environtment Dir"() -> (w382:refnum<vi>)
            n299 = call "element_editor_hydrolysis_initial.vi"("Env. Dir"=w382, "Env. Ready?"=w383, "Break"=w381) -> ()  [unwired: 9 in]
          }
        }
      }
    }
    n300 = local read "Break"() -> (w373:bool)
  }
  n301 = Release Notifier(notifier=w8) -> ()  [unwired: 2 in, 3 out]
  n302 = Merge Errors(w3, w4, w6, w7, w11, w10, w9) -> (w2:errorcluster)
  n303 = call <vilib>:"Clear Errors.vi"("error in (no error)"=w2) -> ()  [unwired: 5 in, 2 out]
